vi "Round 1.vi"(8 "error in (no error)":errorcluster, 11 "KNR in":T1) -> (0 "error out":errorcluster, 3 "KNR out":T1)   [LabVIEW 2013]
uses:
  <userlib>/KNR OS 3.0 LabVIEW Toolkit/Type Definition/KNR3 Reference.ctl
  <userlib>/_FPGA Interface Advanced Tools/FPGA Interface Base/FPGA Interface Base.lvclass
  <userlib>/KNR OS 3.0 LabVIEW Toolkit/Type Definition/Resource.ctl
  <userlib>/KNR OS 3.0 LabVIEW Toolkit/Type Definition/DC Motor Port.ctl
  Global 1.vi
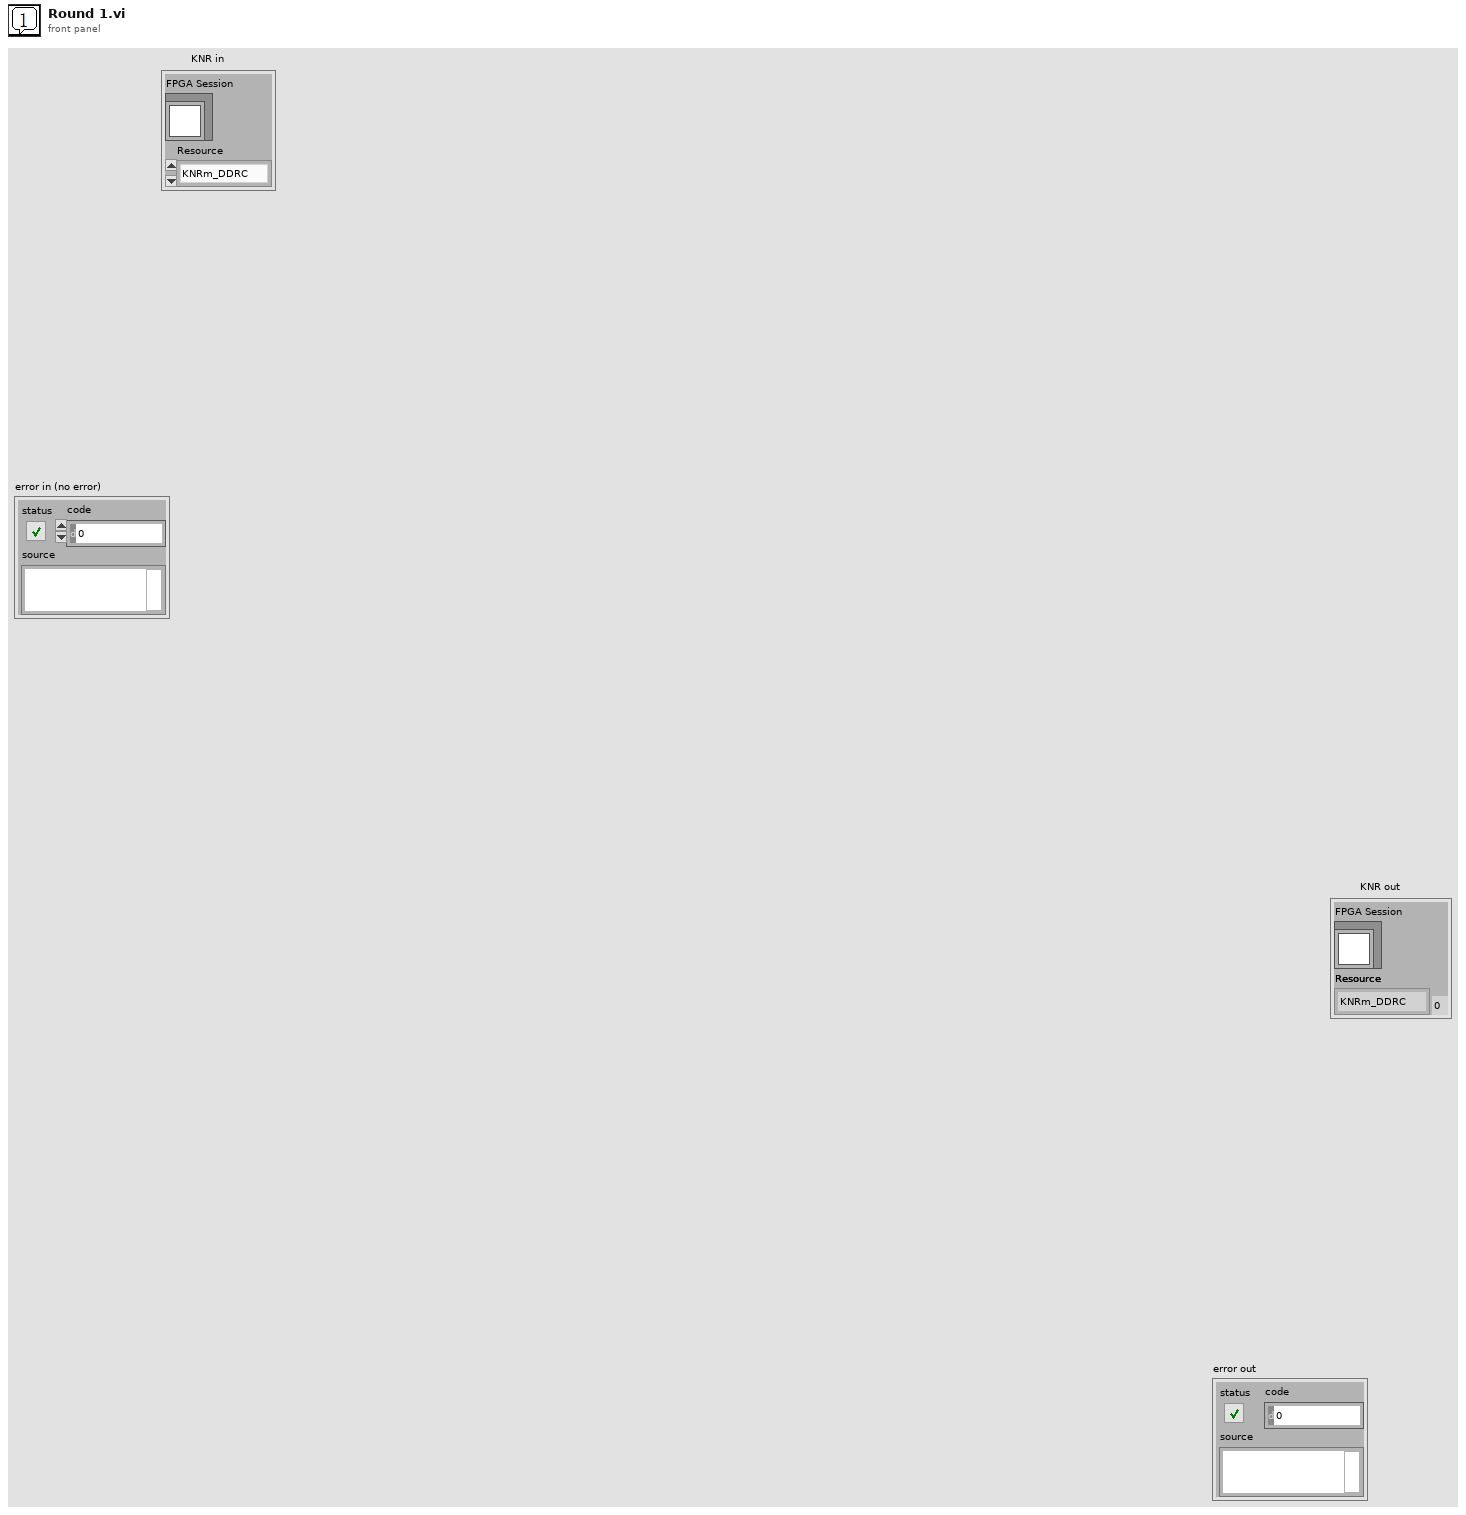
[diagram p1: front panel]
types:
  T1 = typedef "KNR3 Reference.ctl" = cluster{"FPGA Session":refnum<class "FPGA Interface Base.lvclass">, "Resource":T2}
  T2 = typedef "Resource.ctl" = enum16{"KNRm_DDRC", "KNRm_DDDD", "KNRm_DDDR", "KNRm_DDDC", "KNR"}
  T3 = typedef "DC Motor Port.ctl" = u16
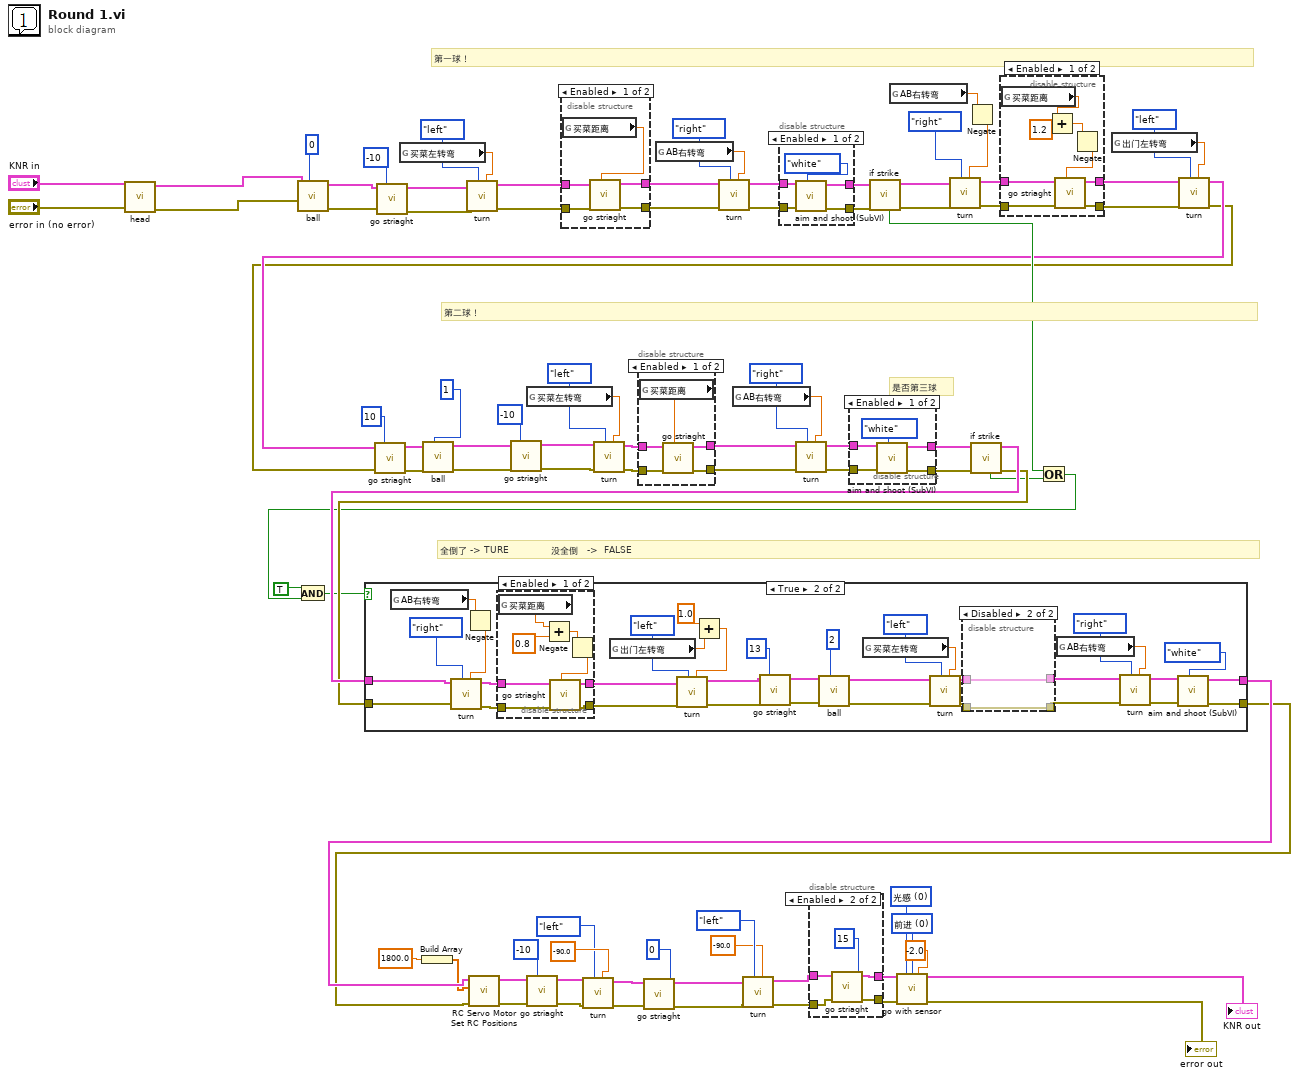
[diagram p0: block diagram]
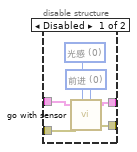
[diagram p2: hidden frame]
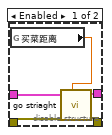
[diagram p9: hidden frame]
diagram:
  w26 = T3 0 items=["前进", "后退"] ("方向")
  w27 = T3 0 items=["光感", "超声波"] ("传感器类型")
  # "是否第三球"
  # "全倒了 -> TURE              没全倒   ->  FALSE"
  # "第二球！"
  # "第一球！"
  n1 = call "head.vi"("error in (no error)"="error in (no error)", "KNR in"="KNR in") -> ("error out"=w1:errorcluster, "KNR out"=w2:T1)  [unwired: 8 in]
  n2 = call "ball.vi"("Numeric"=0, "error in (no error)"=w1, "KNR in"=w2) -> ("error out"=w41:errorcluster, "KNR out"=w42:T1)  [unwired: 6 in, 1 out]
  n3 = call "go striaght.vi"("距离"=-10, "error in (no error)"=w41, "KNR in"=w42) -> ("error out"=w39:errorcluster, "KNR out"=w40:T1)  [unwired: 7 in]
  n4 = global read "Global 1.vi" "买菜左转弯"() -> (w86:dbl)
  n5 = Build Array(1800.0 ("element")) -> (w56:dbl[])
  n6 = call "turn.vi"("Angle"=w86, "side"=enum16{"right", "left"}."left", "error in (no error)"=w39, "KNR in"=w40) -> ("error out"=w87:errorcluster, "KNR out"=w88:T1)  [unwired: 6 in]
  n7 = global read "Global 1.vi" "买菜左转弯"() -> (w69:dbl)
  n8 = disable-structure shown="Enabled" {
    disable-tunnel: w88 -> [w95 w97]
    disable-tunnel: w87 -> [w94 w96]
    disable-tunnel: [w92 w97] -> w83
    disable-tunnel: [w91 w96] -> w82
    frame Enabled {
      n9 = global read "Global 1.vi" "买菜距离"() -> (w93:dbl)
      n10 = call "go striaght.vi"("距离"=w93, "error in (no error)"=w94, "KNR in"=w95) -> ("error out"=w91:errorcluster, "KNR out"=w92:T1)  [unwired: 7 in]
    }
    frame Disabled {
    }
  }
  n11 = global read "Global 1.vi" "AB右转弯"() -> (w85:dbl)
  n12 = call "turn.vi"("Angle"=w85, "side"=enum16{"right", "left"}."right", "error in (no error)"=w82, "KNR in"=w83) -> ("error out"=w49:errorcluster, "KNR out"=w45:T1)  [unwired: 6 in]
  n13 = global read "Global 1.vi" "AB右转弯"() -> (w68:dbl)
  n14 = disable-structure shown="Enabled" {
    disable-tunnel: [w102 w103] -> w54
    disable-tunnel: w49 -> [w101 w103]
    disable-tunnel: w45 -> [w100 w104]
    disable-tunnel: [w99 w104] -> w44
    frame Enabled {
      n15 = call "aim and shoot (SubVI).vi"("pin"=enum16{"white", "green"}."white", "error in (no error)"=w101, "KNR in"=w100) -> ("error out"=w102:errorcluster, "KNR out"=w99:T1)  [unwired: 7 in]
    }
    frame Disabled {
    }
  }
  n16 = call "if strike.vi"("error in (no error)"=w54, "KNR in"=w44) -> ("error out"=w50:errorcluster, "KNR out"=w51:T1, "is strike?"=w53:bool)  [unwired: 7 in]
  n17 = global read "Global 1.vi" "AB右转弯"() -> (w81:dbl)
  n18 = Negate(x=w81) -> (-x=w79:dbl)
  n19 = call "turn.vi"("Angle"=w79, "side"=enum16{"right", "left"}."right", "error in (no error)"=w50, "KNR in"=w51) -> ("error out"=w77:errorcluster, "KNR out"=w78:T1)  [unwired: 6 in]
  n20 = disable-structure shown="Enabled" {
    disable-tunnel: w78 -> [w112 w114]
    disable-tunnel: w77 -> [w111 w113]
    disable-tunnel: [w109 w114] -> w75
    disable-tunnel: [w108 w113] -> w74
    frame Enabled {
      n21 = global read "Global 1.vi" "买菜距离"() -> (w106:dbl)
      n22 = Add(x=w106, y=1.2) -> (x+y=w105:dbl)
      n23 = Negate(x=w105) -> (-x=w110:dbl)
      n24 = call "go striaght.vi"("距离"=w110, "error in (no error)"=w111, "KNR in"=w112) -> ("error out"=w108:errorcluster, "KNR out"=w109:T1)  [unwired: 7 in]
    }
    frame Disabled {
    }
  }
  n25 = global read "Global 1.vi" "出门左转弯"() -> (w46:dbl)
  n26 = call "turn.vi"("Angle"=w46, "side"=enum16{"right", "left"}."left", "error in (no error)"=w74, "KNR in"=w75) -> ("error out"=w7:errorcluster, "KNR out"=w8:T1)  [unwired: 6 in]
  n27 = call "go striaght.vi"("距离"=10, "error in (no error)"=w7, "KNR in"=w8) -> ("error out"=w36:errorcluster, "KNR out"=w37:T1)  [unwired: 7 in]
  n28 = call "ball.vi"("Numeric"=1, "error in (no error)"=w36, "KNR in"=w37) -> ("error out"=w32:errorcluster, "KNR out"=w34:T1)  [unwired: 6 in, 1 out]
  n29 = call "go striaght.vi"("距离"=-10, "error in (no error)"=w32, "KNR in"=w34) -> ("error out"=w31:errorcluster, "KNR out"=w33:T1)  [unwired: 7 in]
  n30 = call "turn.vi"("Angle"=w69, "side"=enum16{"right", "left"}."left", "error in (no error)"=w31, "KNR in"=w33) -> ("error out"=w70:errorcluster, "KNR out"=w71:T1)  [unwired: 6 in]
  n31 = disable-structure shown="Enabled" {
    disable-tunnel: w71 -> [w119 w121]
    disable-tunnel: w70 -> [w118 w120]
    disable-tunnel: [w116 w121] -> w66
    disable-tunnel: [w115 w120] -> w65
    frame Enabled {
      n32 = global read "Global 1.vi" "买菜距离"() -> (w117:dbl)
      n33 = call "go striaght.vi"("距离"=w117, "error in (no error)"=w118, "KNR in"=w119) -> ("error out"=w115:errorcluster, "KNR out"=w116:T1)  [unwired: 7 in]
    }
    frame Disabled {
    }
  }
  n34 = call "turn.vi"("Angle"=w68, "side"=enum16{"right", "left"}."right", "error in (no error)"=w65, "KNR in"=w66) -> ("error out"=w47:errorcluster, "KNR out"=w48:T1)  [unwired: 6 in]
  n35 = disable-structure shown="Enabled" {
    disable-tunnel: [w125 w128] -> w64
    disable-tunnel: [w126 w127] -> w63
    disable-tunnel: w48 -> [w124 w128]
    disable-tunnel: w47 -> [w123 w127]
    frame Enabled {
      n36 = call "aim and shoot (SubVI).vi"("pin"=enum16{"white", "green"}."white", "error in (no error)"=w123, "KNR in"=w124) -> ("error out"=w126:errorcluster, "KNR out"=w125:T1)  [unwired: 7 in]
    }
    frame Disabled {
    }
  }
  n37 = call "if strike.vi"("error in (no error)"=w63, "KNR in"=w64) -> ("error out"=w61:errorcluster, "KNR out"=w62:T1, "is strike?"=w52:bool)  [unwired: 7 in]
  n38 = Or(x=w53, y=w52) -> (x .or. y?=w28:bool)
  n39 = And(x=TRUE, y=w28) -> (x .and. y?=w29:bool)
  n40 = case shown="True" w29 {
    tunnel: w62 -> [w130 w145]
    tunnel: w61 -> [w129 w144]
    tunnel: [w130 w147] -> w58
    tunnel: [w129 w146] -> w57
    frame False {
    }
    frame True {
      n41 = global read "Global 1.vi" "AB右转弯"() -> (w164:dbl)
      n42 = Negate(x=w164) -> (-x=w162:dbl)
      n43 = call "turn.vi"("Angle"=w162, "side"=enum16{"right", "left"}."right", "error in (no error)"=w144, "KNR in"=w145) -> ("error out"=w160:errorcluster, "KNR out"=w161:T1)  [unwired: 6 in]
      n44 = disable-structure shown="Enabled" {
        disable-tunnel: w161 -> [w179 w180]
        disable-tunnel: w160 -> [w178 w181]
        disable-tunnel: [_ w180] -> _
        disable-tunnel: [w176 w181] -> w159
        disable-tunnel: [w172 w180] -> w131
        frame Enabled {
          n45 = global read "Global 1.vi" "买菜距离"() -> (w174:dbl)
          n46 = Add(x=w174, y=0.8) -> (x+y=w173:dbl)
          n47 = Negate(x=w173) -> (-x=w177:dbl)
          n48 = call "go striaght.vi"("距离"=w177, "error in (no error)"=w178, "KNR in"=w179) -> ("error out"=w176:errorcluster, "KNR out"=w172:T1)  [unwired: 7 in]
        }
        frame Disabled {
        }
      }
      n49 = global read "Global 1.vi" "出门左转弯"() -> (w140:dbl)
      n50 = Add(x=1.0, y=w140) -> (x+y=w138:dbl)
      n51 = call "turn.vi"("Angle"=w138, "side"=enum16{"right", "left"}."left", "error in (no error)"=w159, "KNR in"=w131) -> ("error out"=w132:errorcluster, "KNR out"=w133:T1)  [unwired: 6 in]
      n52 = call "go striaght.vi"("距离"=13, "error in (no error)"=w132, "KNR in"=w133) -> ("error out"=w134:errorcluster, "KNR out"=w135:T1)  [unwired: 7 in]
      n53 = call "ball.vi"("Numeric"=2, "error in (no error)"=w134, "KNR in"=w135) -> ("error out"=w155:errorcluster, "KNR out"=w156:T1)  [unwired: 6 in, 1 out]
      n54 = global read "Global 1.vi" "买菜左转弯"() -> (w152:dbl)
      n55 = call "turn.vi"("Angle"=w152, "side"=enum16{"right", "left"}."left", "error in (no error)"=w155, "KNR in"=w156) -> ("error out"=w153:errorcluster, "KNR out"=w154:T1)  [unwired: 6 in]
      n56 = disable-structure shown="Disabled" {
        disable-tunnel: w154 -> [w169 w171]
        disable-tunnel: w153 -> [w168 w170]
        disable-tunnel: [w166 w171] -> w149
        disable-tunnel: [w165 w170] -> w148
        frame Enabled {
          n57 = global read "Global 1.vi" "买菜距离"() -> (w167:dbl)
          n58 = call "go striaght.vi"("距离"=w167, "error in (no error)"=w168, "KNR in"=w169) -> ("error out"=w165:errorcluster, "KNR out"=w166:T1)  [unwired: 7 in]
        }
        frame Disabled {
        }
      }
      n59 = global read "Global 1.vi" "AB右转弯"() -> (w151:dbl)
      n60 = call "turn.vi"("Angle"=w151, "side"=enum16{"right", "left"}."right", "error in (no error)"=w148, "KNR in"=w149) -> ("error out"=w142:errorcluster, "KNR out"=w143:T1)  [unwired: 6 in]
      n61 = call "aim and shoot (SubVI).vi"("pin"=enum16{"white", "green"}."white", "error in (no error)"=w142, "KNR in"=w143) -> ("error out"=w146:errorcluster, "KNR out"=w147:T1)  [unwired: 7 in]
    }
  }
  n62 = call <userlib>:"RC Servo Motor Set RC Positions.vi"("error in (no error)"=w57, "RC Pulse Width (1500 uS)"=w56, "KNR in"=w58) -> ("error out"=w18:errorcluster, "KNR out"=w19:T1)  [unwired: 7 in]
  n63 = call "go striaght.vi"("距离"=-10, "error in (no error)"=w18, "KNR in"=w19) -> ("error out"=w20:errorcluster, "KNR out"=w21:T1)  [unwired: 7 in]
  n64 = call "turn.vi"("Angle"=-90.0, "side"=enum16{"right", "left"}."left", "error in (no error)"=w20, "KNR in"=w21) -> ("error out"=w15:errorcluster, "KNR out"=w16:T1)  [unwired: 6 in]
  n65 = call "go striaght.vi"("距离"=0, "error in (no error)"=w15, "KNR in"=w16) -> ("error out"=w11:errorcluster, "KNR out"=w12:T1)  [unwired: 7 in]
  n66 = call "turn.vi"("Angle"=-90.0, "side"=enum16{"right", "left"}."left", "error in (no error)"=w11, "KNR in"=w12) -> ("error out"=w9:errorcluster, "KNR out"=w10:T1)  [unwired: 6 in]
  n67 = disable-structure shown="Enabled" {
    disable-tunnel: [w185 w191] -> w24
    disable-tunnel: [w184 w190] -> w23
    disable-tunnel: w10 -> [w183 w189]
    disable-tunnel: w9 -> [w182 w188]
    frame Disabled {
      w186 = T3 0 items=["前进", "后退"] ("方向")
      w187 = T3 0 items=["光感", "超声波"] ("传感器类型")
      n68 = call "go with sensor.vi"("KNR in"=w183, "传感器类型"=w187, "error in (no error)"=w182, "方向"=w186) -> ("KNR out"=w185:T1, "error out"=w184:errorcluster)  [unwired: 3 in, 1 out]
    }
    frame Enabled {
      n69 = call "go striaght.vi"("距离"=15, "error in (no error)"=w188, "KNR in"=w189) -> ("error out"=w190:errorcluster, "KNR out"=w191:T1)  [unwired: 7 in]
    }
  }
  n70 = call "go with sensor.vi"("KNR in"=w24, "传感器类型"=w27, "方向"=w26, "then go:"=-2.0, "error in (no error)"=w23) -> ("KNR out"=→"KNR out":T1, "error out"=→"error out":errorcluster)  [unwired: 8 in, 1 out]
